vi "ParameterSelect.vi"(5 "模式":T1(ring)=enum."selectsave", 7 "productsName":string, 11 "parameterName":string) -> (0 "limitL":dbl=nan, 1 "limitH":dbl=nan, 2 "vaule":dbl=nan, 3 "dataOutAll":string[][](array[string]), 4 "unit":string, 6 "result":string)   [LabVIEW 2012]
uses:
  <vilib>/Utility/VariantDataType/Type.ctl
  <vilib>/Utility/VariantDataType/VariantType.lvlib
panel:
  out "notes":string
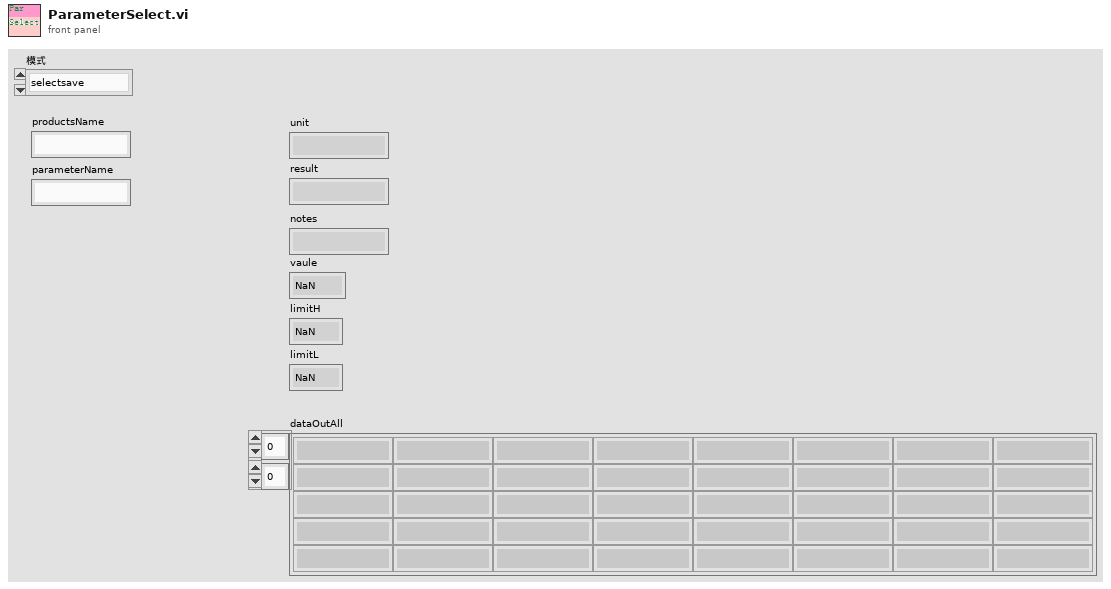
[diagram p1: front panel]
types:
  T1 = enum16{"selectdata", "selectsave", "selectlist", "selectshow"}
  T2 = typedef "VariantType.lvlib/Type.ctl" = enum8{"Invalid Type", "Void", "I8", "I16", "I32", "I64", "U8", "U16", "U32", "U64", "Single Float", "Double Float", "Extended Float", "Single Complex", "Double Complex", "Extended Complex", "Enum U8", "Enum U16", "Enum U32", "Enum U64", "Single Float With Unit", "Double Float With Unit", "Extended Float With Unit", "Single Complex with Unit", "Double Complex with Unit", "Extended Complex with Unit", "Boolean", "String", "Path", "Picture", "Tag", "Array", "Cluster", "Variant", "LV Variant", "Waveform", "Timestamp", "Digital Waveform", "Digital Data", "ExpressData", "Refnum", "External Data", "VI", "Poly VI", "LabVIEW Class Instance", "Fixed Point"}
  T3 = cluster{"Type Enum":T2, "name":string, "data":string}[]
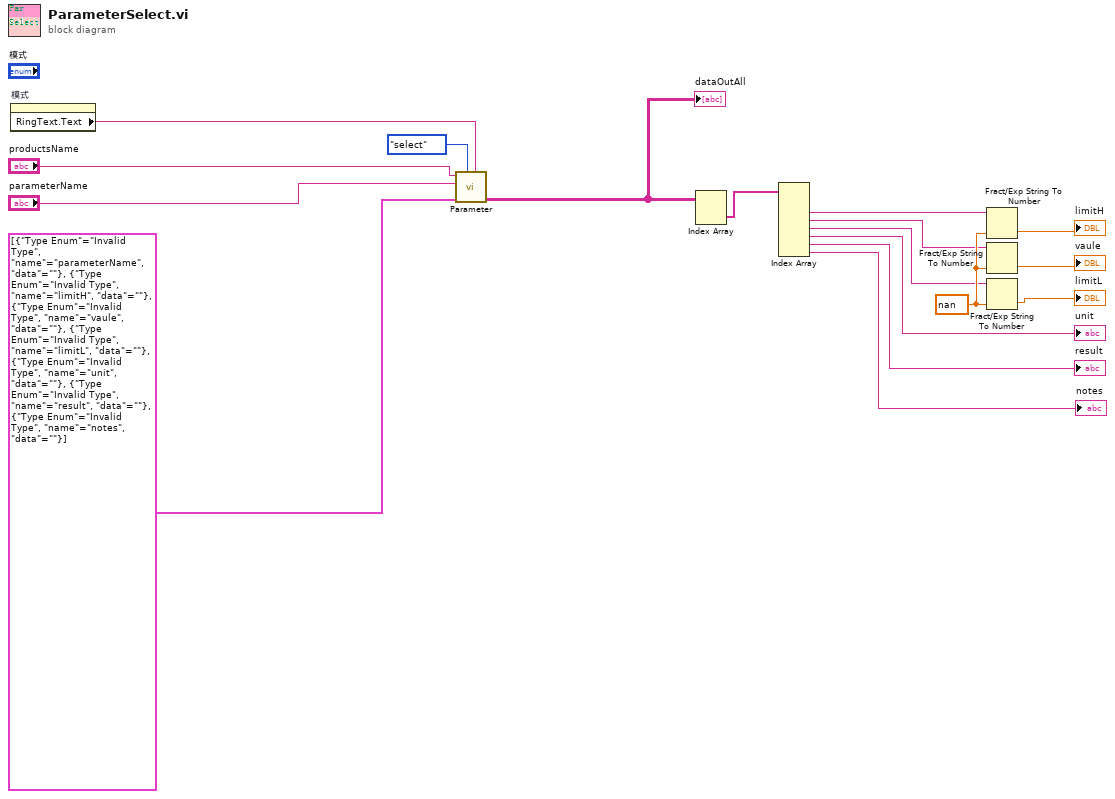
[diagram p0: block diagram]
diagram:
  w12 = nan ("默认(0 DBL)")
  n1 = property on="模式" class="Enum (严格)"() -> ("RingText.Text"=w16:string)  [unwired: 2 in, 2 out]
  n2 = call "Parameter.vi"("继承模式"=w16, "模式"=enum16{"select", "insert", "update", "delete"}."select", "nameData"=T3 [{"Type Enum"=enum."Invalid Type", "name"="parameterName", "data"=""}, {"Type Enum"=enum."Invalid Type", "name"="limitH", "data"=""}, {"Type Enum"=enum."Invalid Type", "name"="vaule", "data"=""}, {"Type Enum"=enum."Invalid Type", "name"="limitL", "data"=""}, {"Type Enum"=enum."Invalid Type", "name"="unit", "data"=""}, {"Type Enum"=enum."Invalid Type", "name"="result", "data"=""}, {"Type Enum"=enum."Invalid Type", "name"="notes", "data"=""}], "parameterName"="parameterName", "productsName"="productsName") -> ("data"=w3:string[][])  [unwired: 6 in]
  "dataOutAll" <- w3
  n3 = Index Array(array=w3) -> (element=w2:string[])  [unwired: 2 in]
  n4 = Index Array(array=w2) -> (element #2=w11:string, element #3=w10:string, element #4=w9:string, element #5=→"unit":string, element #6=→"result":string, element #7=→"notes":string)  [unwired: 7 in, 1 out]
  n5 = Fract/Exp String To Number(string=w11, default (0 dbl)=w12) -> (number=→"limitH":dbl)  [unwired: 2 in, 1 out]
  n6 = Fract/Exp String To Number(string=w10, default (0 dbl)=w12) -> (number=→"vaule":dbl)  [unwired: 2 in, 1 out]
  n7 = Fract/Exp String To Number(string=w9, default (0 dbl)=w12) -> (number=→"limitL":dbl)  [unwired: 2 in, 1 out]
